vi "State_Machine.vi"(8 "error in (no error)":errorcluster caption="entrée d'erreur (pas d'erreur)", 11 "Flash_Jlink en entrée":refnum<class "P2265_Boot_IEEE.lvclass">) -> (0 "error out":errorcluster caption="sortie d'erreur", 2 "Json_String":string, 3 "Flash_Jlink en sortie":refnum<class "P2265_Boot_IEEE.lvclass">)   [LabVIEW 2020, in "Library Test.lvlib" / "P2265_Boot_IEEE.lvclass"]
uses:
  P2265_Boot_IEEE.lvclass
  Process/Process (Default)/Process (Default).lvclass
  <vilib>/Platform/TimedLoop/XDataNode/timing_clust.ctl
  <vilib>/Platform/TimedLoop/XDataNode/nitl_modes.ctl
  <vilib>/Platform/TimedLoop/XDataNode/wakeup.ctl
  JSON API/Variant JSON/Variant to JSON.vi
  JSON API/JSON Value/Get Item by name array.vi
  <vilib>/Platform/TimedLoop/XDataNode/XDataNode.xnode
  JSON API/JSON Value/JSON Value.lvclass
  P2265_Boot_IEEE.lvclass/P2265_Boot_IEEE.ctl
  <vilib>/Platform/TimedLoop/XDataNode/XDNodeRunTimeDep.lvlib
  JSON API/Get Polymorphic/JSON GetSet.lvlib
  Commun VI/Library Commun.lvlib
  JSON API/Variant JSON/Variant JSON.lvlib
panel:
  out "String In progress":string
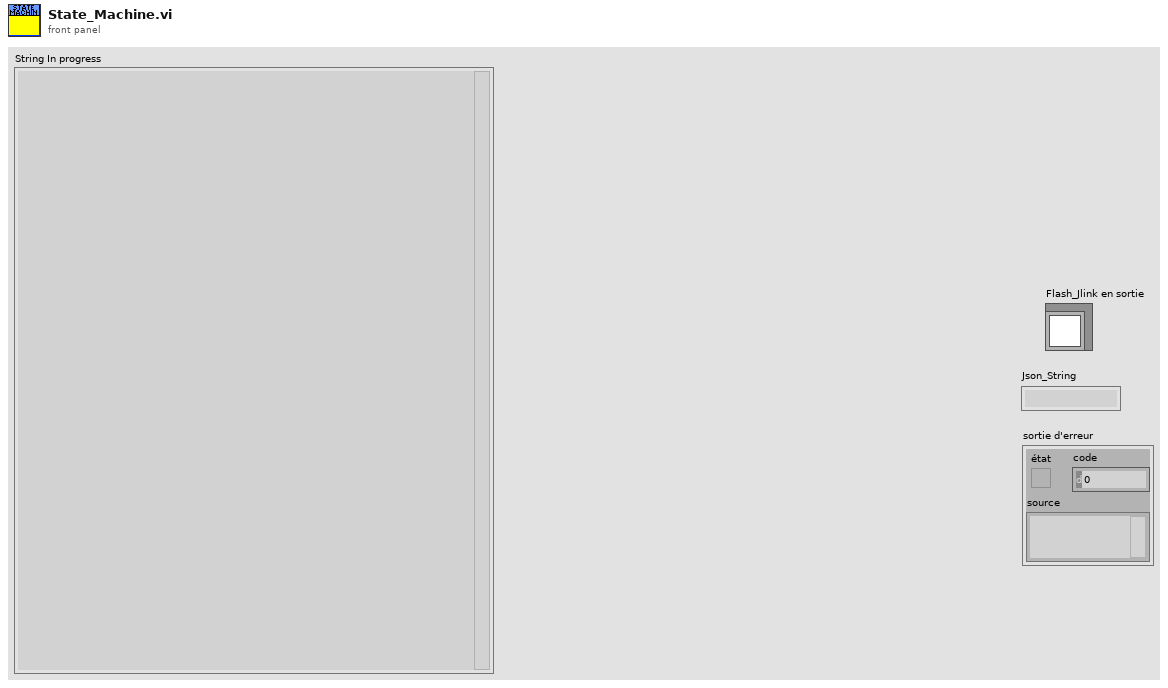
[diagram p1: front panel]
types:
  T1 = cluster{"FW Version":string, "IEE Address":string}
  T2 = typedef "XDNodeRunTimeDep.lvlib/timing_clust.ctl" = cluster{"Expected End [f-1]":u64, "Actual End [f-1]":u64, "Finished Late? [f-1]":bool, "Expected End [i-1]":u64, "Actual End [i-1]":u64, "Finished Late? [i-1]":bool, "Expected Start [i]":u64, "Actual Start [i]":u64, "Expected Start [f]":u64, "Actual Start [f]":u64, "Source Name":string, "Structure Name":string, "Period":i64, "Deadline":i64, "Offset":i64, "Start":i64, "Priority":i32, "Timeout":i32, "Mode":T3, "Wakeup Reason":T4, "Error":errorcluster, "Source Type":string, "Secondary Source Type":string, "Global End Time":u64, "Global Start Time":u64, "Frame Duration":u64, "Iteration Duration":u64, "Assigned CPU":i32, "I/O Scan Engine Mode":u32}
  T3 = typedef "XDNodeRunTimeDep.lvlib/nitl_modes.ctl" = enum32{"No Change", "Process missed periods, maintain original phase", "Discard missed periods, maintain original phase", "Process missed periods, ignore original phase", "Discard missed periods, ignore original phase"}
  T4 = typedef "XDNodeRunTimeDep.lvlib/wakeup.ctl" = enum32{"Normal", "Aborted", "Asynchronous wakeup", "Timing source error", "Timed loop error", "Timeout"}
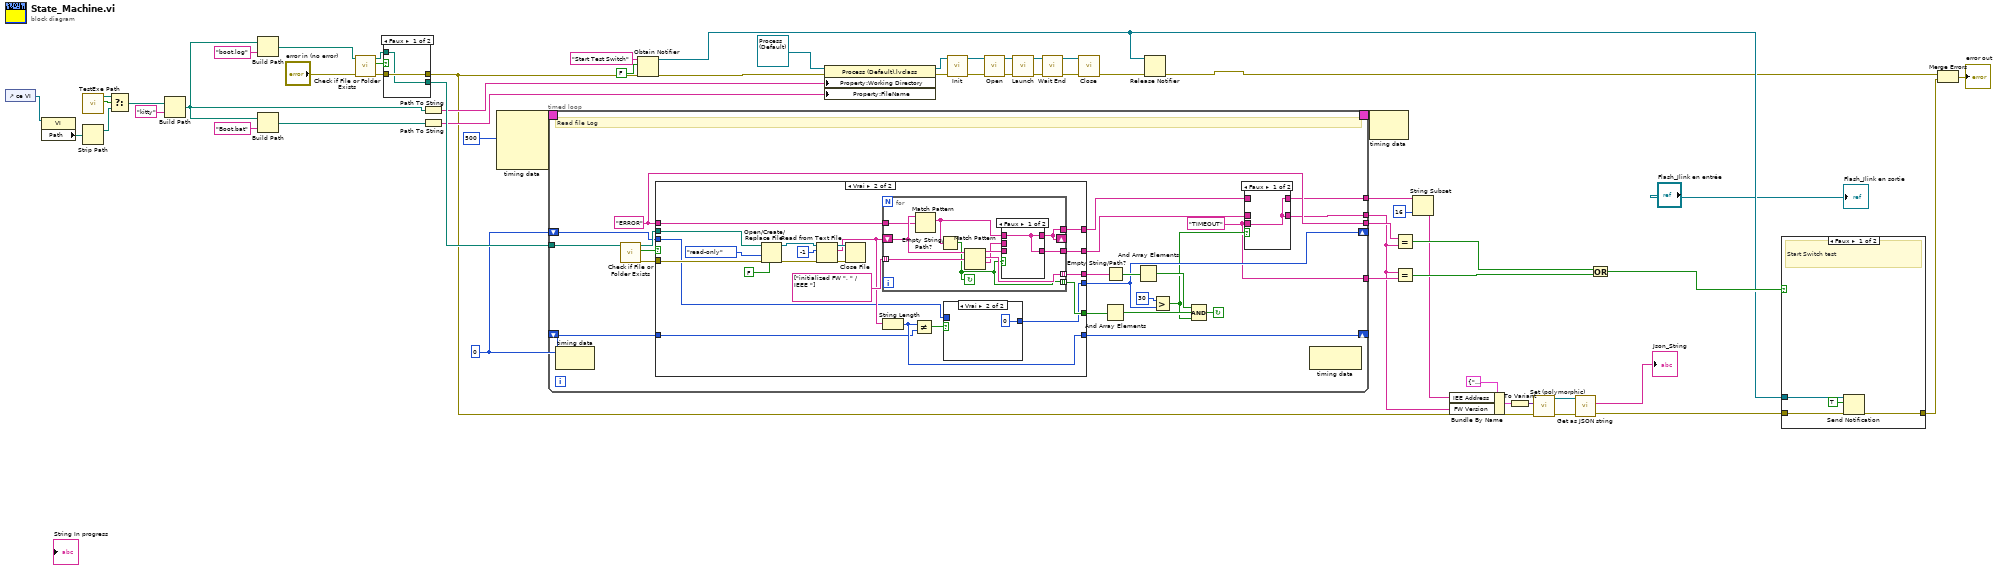
[diagram p0: block diagram]
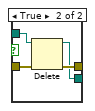
[diagram p2: hidden frame]
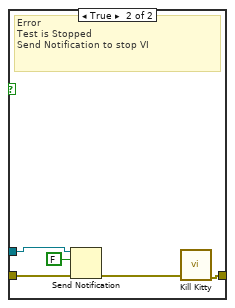
[diagram p3: hidden frame]
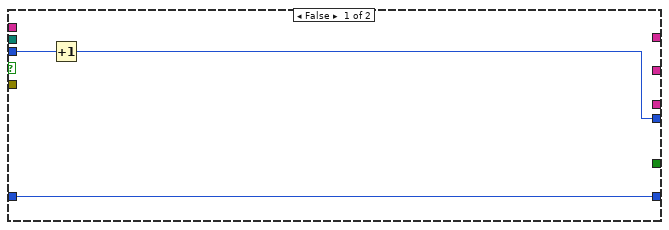
[diagram p5: hidden frame]
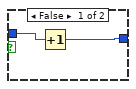
[diagram p6: hidden frame]
diagram:
  w29 = 0
  n1 = control-ref of="ce VI"() -> (w60:refnum<vi>)
  n2 = property class="VI"(reference=w60) -> ("Path"=w59:path)  [unwired: 1 in, 2 out]
  n3 = call "TestExe Path.vi"() -> ("En Exe?"=w4:bool, "Chemin Actuel"=w5:path)  [unwired: 9 in, 1 out]
  n4 = Strip Path(path=w59) -> (stripped path=w1:path)  [unwired: 1 out]
  n5 = Select(t=w5, s=w4, f=w1) -> (s? t:f=w3:path)
  n6 = Build Path(base path=w3, name or relative path="kitty" ("nom ou chemin relatif")) -> (appended path=w2:path)
  n7 = Build Path(base path=w2, name or relative path="boot.log" ("nom ou chemin relatif")) -> (appended path=w55:path)
  n8 = Build Path(base path=w2, name or relative path="Boot.bat" ("nom ou chemin relatif")) -> (appended path=w35:path)
  n9 = call <vilib>:"Check if File or Folder Exists.vi"("error in (no error)"="error in (no error)", "path"=w55) -> ("error out"=w46:errorcluster, "file or folder exists?"=w45:bool, "dup path"=w31:path)  [unwired: 7 in]
  n10 = case shown="Faux" w45 {
    tunnel: [w62 w66] -> w12
    tunnel: [w61 w65] -> w47
    tunnel: w31 -> [w61 w64]
    tunnel: w46 -> [w62 w63]
    frame False {
    }
    frame True {
      n11 = Delete(path (use dialog)=w64, error in=w63) -> (deleted path=w65:path, error out=w66:errorcluster)  [unwired: 3 in, 1 out]
    }
  }
  n12 = Path To String(path=w2) -> (string=w36:string)
  n13 = Path To String(path=w35) -> (string=w30:string)
  n14 = node-c288(i64 500 ("Période")) -> (w54:T2)  [unwired: 3 in]
  n15 = timed-loop {
    tunnel: w47 -> [w88]
    timing: w54 -> [_]
    timing-out: [_] -> w53
    tunnel: [w68] -> w10
    tunnel: [w70] -> w13
    tunnel: [w78] -> w48
    shift-right: [w77] -> _
    shift-left: w29 -> [w76]
    shift-right: [w74] -> _
    shift-left: w29 -> [w75]
    tunnel: [w67] -> w25
    stop <- w81 continue-if-true
    w67 = "TIMEOUT" ("expression régulière")
    w78 = "ERROR" ("expression régulière")
    # "Read file Log"
    n16 = node-c288() -> ()  [unwired: 1 in, 1 out]
    n17 = call <vilib>:"Check if File or Folder Exists.vi"("path"=w88) -> ("error out"=w85:errorcluster, "file or folder exists?"=w86:bool, "dup path"=w87:path)  [unwired: 8 in]
    n18 = case shown="Vrai" w86 {
      tunnel: w87 -> [_ w113]
      tunnel: w85 -> [_ w110]
      tunnel: [_ w106] -> w69
      tunnel: [_ w105] -> w71
      tunnel: [_ w103] -> w84
      tunnel: [_ w102] -> w82
      tunnel: w78 -> [_ w101]
      tunnel: [w94 w97] -> w77
      tunnel: w76 -> [w94 w96]
      tunnel: w75 -> [w93 w99]
      tunnel: [w92 w98] -> w74
      frame False {
        n19 = Increment(x=w93) -> (x+1=w92:i32)
      }
      frame True {
        n20 = Open/Create/Replace File(file path (use dialog)=w113, error in=w110, access (0:read/write)=enum16{"read/write", "read-only", "write-only"}."read-only" ("accès (0 : read/write)"), disable buffering (F)=FALSE ("désactiver la bufférisation (F)")) -> (refnum out=w112:refnum<file>, error out=w111:errorcluster)  [unwired: 2 in, 1 out]
        n21 = Read from Text File(file (use dialog)=w112, count=-1 ("nombre"), error in=w111) -> (refnum out=w108:refnum<file>, text=w100:string, error out=w109:errorcluster)  [unwired: 1 in, 1 out]
        n22 = Close File(refnum=w108, error in=w109) -> ()  [unwired: 2 out]
        n23 = for {
          tunnel: string[] ["initialized FW ", " / IEEE "] -> [w128] mode=indexing
          tunnel: [w124] -> w106
          tunnel: [w122] -> w105
          tunnel: [w127] -> w103 mode=indexing
          shift-right: [w122] -> _
          shift-left: w100 -> [w126]
          tunnel: [w120] -> w102 mode=indexing
          tunnel: w101 -> [w119]
          stop <- w120 continue-if-true
          n24 = Match Pattern(string=w126, regular expression=w119) -> (match substring=w121:string)  [unwired: 1 in, 3 out]
          n25 = Empty String/Path?(string/path=w121) -> (empty?=w120:bool)
          n26 = Match Pattern(string=w126, regular expression=w128) -> (before substring=w125:string, match substring=w127:string, after substring=w123:string)  [unwired: 1 in, 1 out]
          n27 = case shown="Faux" w120 {
            tunnel: w125 -> [_ w131]
            tunnel: [w129 w131] -> w124
            tunnel: [w129 w130] -> w122
            tunnel: w123 -> [_ w130]
            tunnel: w121 -> [w129 _]
            frame False {
            }
            frame True {
            }
          }
        }
        n28 = String Length(string=w100) -> (length=w97:i32)
        n29 = Not Equal?(x=w97, y=w96) -> (x != y?=w95:bool)
        n30 = case shown="Vrai" w95 {
          tunnel: w99 -> [w117 _]
          tunnel: [w116 0] -> w98
          frame False {
            n31 = Increment(x=w117) -> (x+1=w116:i32)
          }
          frame True {
          }
        }
      }
    }
    n32 = Empty String/Path?(string/path=w84) -> (empty?=w83:bool[])
    n33 = And Array Elements(Boolean array=w82) -> (logical AND=w79:bool)
    n34 = And Array Elements(Boolean array=w83) -> (logical AND=w80:bool)
    n35 = Greater?(x=30, y=w74) -> (0:w72:bool)
    n36 = Compound Arithmetic op=AND ("Opérateur arithmétique")(w80, w79, w72) -> (w81:bool)
    n37 = case shown="Faux" w72 {
      tunnel: w67 -> [w89 _]
      tunnel: w71 -> [_ w90]
      tunnel: [w89 w90] -> w70
      tunnel: w69 -> [_ w91]
      tunnel: [w89 w91] -> w68
      frame False {
      }
      frame True {
      }
    }
    n38 = node-c288() -> ()  [unwired: 1 in, 1 out]
  }
  n39 = Obtain Notifier(name (unnamed)="Start Test Switch" ("nom (aucun)"), notification data type=FALSE, error in (no error)=w12) -> (notifier out=w19:refnum<notifier>, error out=w23:errorcluster)  [unwired: 1 in, 1 out]
  n40 = property class="Process (Default).lvclass"(reference=refnum<class "Process (Default).lvclass"> refnum ("Process (Default).lvclass"), error in=w23, "Property:Working Directory"=w36, "Property:FileName"=w30) -> (reference out=w42:refnum<class "Process (Default).lvclass">, error out=w24:errorcluster)
  n41 = call-dynamic "Init.vi"("error in (no error)"=w24, "Process (Default) en entrée"=w42) -> ("error out"=w41:errorcluster, "Process (Default) en sortie"=w40:refnum<class "Process (Default).lvclass">)  [unwired: 8 in]
  n42 = call-dynamic "Open.vi"("error in (no error)"=w41, "Process (Default) en entrée"=w40) -> ("error out"=w39:errorcluster, "Process (Default) en sortie"=w38:refnum<class "Process (Default).lvclass">)  [unwired: 8 in]
  n43 = call-dynamic "Launch.vi"("error in (no error)"=w39, "Process (Default) en entrée"=w38) -> ("error out"=w33:errorcluster, "Process (Default) en sortie"=w32:refnum<class "Process (Default).lvclass">)  [unwired: 8 in]
  n44 = call-dynamic "Wait End.vi"("error in (no error)"=w33, "Process (Default) en entrée"=w32) -> ("error out"=w44:errorcluster, "Process (Default) en sortie"=w43:refnum<class "Process (Default).lvclass">)  [unwired: 8 in]
  n45 = call-dynamic "Close.vi"("error in (no error)"=w44, "Process (Default) en entrée"=w43) -> ("error out"=w20:errorcluster)  [unwired: 8 in, 1 out]
  n46 = Release Notifier(notifier=w19, error in (no error)=w20) -> (error out=w11:errorcluster)  [unwired: 1 in, 2 out]
  n47 = node-c288(w53) -> ()  [unwired: 1 out]
  n48 = Equal?(x=w48, y=w10) -> (x = y?=w27:bool)
  n49 = Equal?(x=w10, y=w25) -> (x = y?=w28:bool)
  n50 = String Subset(string=w13, length (rest)=16 ("longueur (reste)")) -> (substring=w9:string)  [unwired: 1 in]
  n51 = Bundle By Name(cluster=T1 {"FW Version"="", "IEE Address"=""} ("Cluster des données privées de classe"), "IEE Address"=w9, "FW Version"=w10) -> (w14:T1)
  n52 = To Variant(anything=w14) -> (Variant=w18:variant)
  n53 = call-poly "Set (polymorphic).vi"("error in (no error)"=w12, "Variant"=w18) -> ("error out"=w16:errorcluster, "JSON Value out"=w17:refnum<class "JSON Value.lvclass">)  [unwired: 8 in]
  n54 = call "Get as JSON string.vi"("error in (no error)"=w16, "JSON Value in"=w17) -> ("error out"=w6:errorcluster, "<JSON>"=→"Json_String":string)  [unwired: 8 in]
  n55 = Or(x=w27, y=w28) -> (x .or. y?=w26:bool)
  n56 = case shown="Faux" w26 {
    tunnel: w6 -> [w137 w141]
    tunnel: [w134 w142] -> w51
    tunnel: w19 -> [w136 w140]
    frame False {
      # "Start Switch test"
      n57 = Send Notification(notification=TRUE, notifier=w136, error in (no error)=w137) -> (error out=w134:errorcluster)  [unwired: 1 out]
    }
    frame True {
      # "Error\nTest is Stopped\nSend Notification to stop VI"
      n58 = Send Notification(notification=FALSE, notifier=w140, error in (no error)=w141) -> (error out=w138:errorcluster)  [unwired: 1 out]
      n59 = call "Kill Kitty.vi"("error in (no error)"=w138) -> ("error out"=w142:errorcluster)  [unwired: 10 in]
    }
  }
  n60 = Merge Errors(w11, w51) -> (→"error out":errorcluster)
  "Flash_Jlink en sortie" <- "Flash_Jlink en entrée"
